vi "Load CHM Page.vi"(8 "error in (no error)":errorcluster, 9 "HTML File":string="MainPage_J1939.html", 10 "Compiled CHM Path":path, 11 "Web Browser Reference":refnum<k7>(container)) -> (0 "error out":errorcluster)   [LabVIEW 2027]
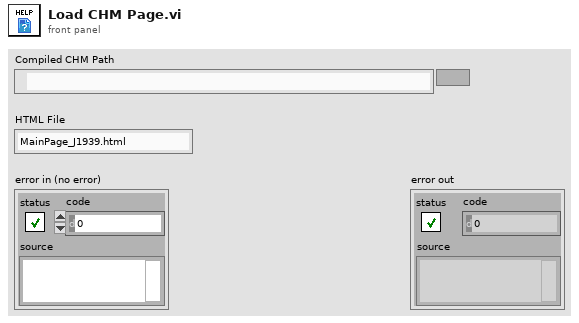
[diagram p1: front panel]
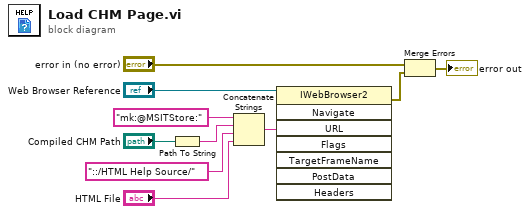
[diagram p0: block diagram]
diagram:
  n1 = Path To String(path="Compiled CHM Path") -> (string=w8:string)
  n2 = Concatenate Strings("mk:@MSITStore:" ("string"), w8, "::/HTML Help Source/" ("name or relative path"), "HTML File") -> (w1:string)
  n3 = invoke class="IWebBrowser2" method="Navigate"(reference="Web Browser Reference", "URL"=w1) -> (error out=w5:errorcluster)  [unwired: 6 in, 7 out]
  n4 = Merge Errors("error in (no error)", w5) -> (→"error out":errorcluster)
